vi "Append Page number HF.vi"(0 "PDF Report IN":refnum<class "PDF Report Class.lvclass">, 2 "Header or footer":T1={"Start at page"=1, "Start with #"=1, "Cell Alignment"=1, "Page #"={"Text 1"="", "Text 2"="", "Text 3"=""}, "Font"={"Name"="", "Size"=-1.0, "Color"=0, "Style"={"Bold"=FALSE, "Italic"=FALSE, "Underline"=FALSE, "Strikeout"=FALSE}, "Type"={"Type&direction"=enum."Select", "Embedded"=FALSE, "Encoding"=""}}}, 11 "error in (no error)":errorcluster, 13 "Position":T9) -> (4 "PDF Report OUT":refnum<class "PDF Report Class.lvclass">, 15 "error out":errorcluster)   [LabVIEW 2019, in "Exaprom PDF.lvlib"]
doc: "Appends a <B>page number</B> in a column header (or footer). You can use this polymorphic VI to append a colomn to a header (or footer). The data type you wire to the <B>Header or footer</B> input determines the polymorphic instance to use.\n\nThe header (or footer) can be divided up into three columns. Each column has the same width. The number of header (or footer) that you add determines the number of columns.\n\n<B>FRANÇAIS</B>\nAjoute un <B>numéro de page</B> dans une colonne d'un en-tête (ou d'un pied de page). Vous pouvez utiliser ce VI polymorphique pour ajouter une colonne à un en-tête (ou un pied de page). Le type de variable que vous reliez au terminal <B>Header or footer</B> détermine l'instance polymorphique à utiliser.\n\nL'en-tête (ou le pied de page) peut être divisé en un maximum de trois colonnes. Chaque colonne a la même largeur. Le nombre d'en-têtes (ou de pieds de page) que vous ajoutez détermine le nombre de colonnes.\n\n\n\nVersion 1.1\nDeveloped by Jean-Marc Simard\nCopyright © 2012, Exaprom Inc.\nAll rights reserved.\nLicense: BSD\n\nWith iTextSharp 4.1.6 (http://itextsharp.sourceforge.net)\nunder Mozilla Public License Version 1.1\n(http://www.mozilla.org/MPL/MPL-1.1.html)"
uses:
  Exaprom PDF.lvlib
  LV Class/PDF Report Class/PDF Report Class.lvclass
  Controls/Header, Footer and Watermark Controls/Header or Footer.ctl
  Controls/Header, Footer and Watermark Controls/Header or Footer  Page # cluster.ctl
  Controls/Table Controls/Cell Alignment 20px.ctl
  Controls/Header, Footer and Watermark Controls/Page number.ctl
  Controls/Font Controls/Font complete cluster horizontal.ctl
  Controls/Font Controls/Font size.ctl
  Controls/Font Controls/Font color.ctl
  Controls/Font Controls/Type and encoding.ctl
  Controls/Text Controls/Unicode/Type and run direction.ctl
  LV Class/Header and Footer Class/VIs/Controls/Header Footer cluster V2.ctl
  Controls/Header, Footer and Watermark Controls/Header Footer Type.ctl
  Controls/Header, Footer and Watermark Controls/Header footer horiz alignment.ctl
  Controls/Table Controls/Cell Vertical alignment.ctl
  Controls/Text Controls/Line spacing.ctl
  Controls/Header, Footer and Watermark Controls/Header Footer Line.ctl
  C:/work/niobrara_lv/labview pdf writer fixing/DLL/itextsharp.dll
  DLL/itextsharp.dll
  LV Class/Fonts Class/Font Class.lvclass
  LV Class/Header and Footer Class/Header and Footer Class.lvclass
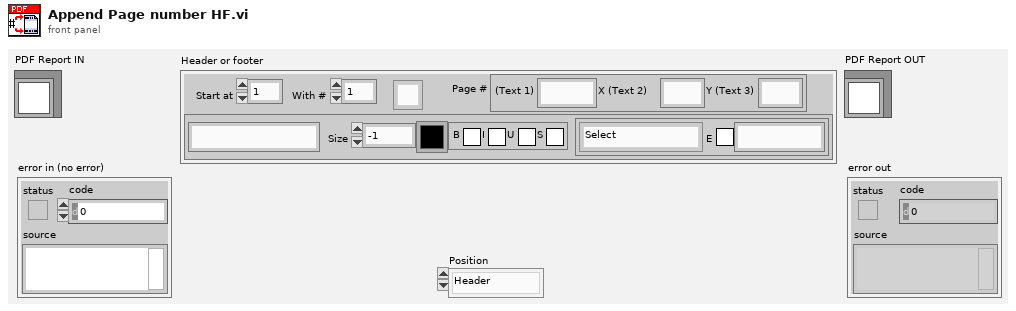
[diagram p1: front panel]
types:
  T1 = typedef "Exaprom PDF.lvlib/Header or Footer  Page # cluster.ctl" = cluster{"Start at page":i32, "Start with #":i32, "Cell Alignment":T2, "Page #":T3, "Font":T4}
  T2 = typedef "Exaprom PDF.lvlib/Cell Alignment 20px.ctl" = u16
  T3 = typedef "Exaprom PDF.lvlib/Page number.ctl" = cluster{"Text 1":string, "Text 2":string, "Text 3":string}
  T4 = typedef "Exaprom PDF.lvlib/Font complete cluster horizontal.ctl" = cluster{"Name":string, "Size":T5, "Color":T6, "Style":cluster{"Bold":bool, "Italic":bool, "Underline":bool, "Strikeout":bool}, "Type":T7}
  T5 = typedef "Exaprom PDF.lvlib/Font size.ctl" = sgl
  T6 = typedef "Exaprom PDF.lvlib/Font color.ctl" = u32
  T7 = typedef "Exaprom PDF.lvlib/Type and encoding.ctl" = cluster{"Type&direction":T8, "Embedded":bool, "Encoding":string}
  T8 = typedef "Exaprom PDF.lvlib/Type and run direction.ctl" = enum16{"Select", "ASCII", "UTF-16", "UTF-16 (default)", "UTF-16 (LTR)", "UTF-16 (RTL)"}
  T9 = typedef "Exaprom PDF.lvlib/Header or Footer.ctl" = enum16{"Header", "Footer"}
  T10 = typedef "Exaprom PDF.lvlib/Header and Footer Class.lvclass/Header Footer cluster V2.ctl" = cluster{"Header or Footer":T9, "Start page":i32, "Start with #":i32, "Type":T11, "Alignment":T12, "Vertical Alignement":T13, "Line spacing":T14, "Image (%)":sgl, "Page #":T3, "Text":string, "Path":string, "Font":T4, "Font refnum":refnum<k24>, "Line":cluster{"Line":T15, "Thickness (points)":sgl, "Colour":T6}, "Vert margin":dbl, "Hyperlink":string}
  T11 = typedef "Exaprom PDF.lvlib/Header Footer Type.ctl" = enum16{"Select", "Text", "Text + hyperlink", "Page number", "Image", "Image + hyperlink"}
  T12 = typedef "Exaprom PDF.lvlib/Header footer horiz alignment.ctl" = enum16{"Left", "Center", "Right"}
  T13 = typedef "Exaprom PDF.lvlib/Cell Vertical alignment.ctl" = enum16{"TOP", "MIDDLE", "BOTTOM"}
  T14 = typedef "Exaprom PDF.lvlib/Line spacing.ctl" = enum16{"Select", "1.0", "1.5", "2.0"}
  T15 = typedef "Exaprom PDF.lvlib/Header Footer Line.ctl" = enum16{"No line", "Horizontal line"}
  T16 = typedef "Exaprom PDF.lvlib/Font complete cluster.ctl" = cluster{"Name":string, "Size":T5, "Color":T6, "Style":cluster{"Bold":bool, "Italic":bool, "Underline":bool, "Strikeout":bool}, "Type":T7}
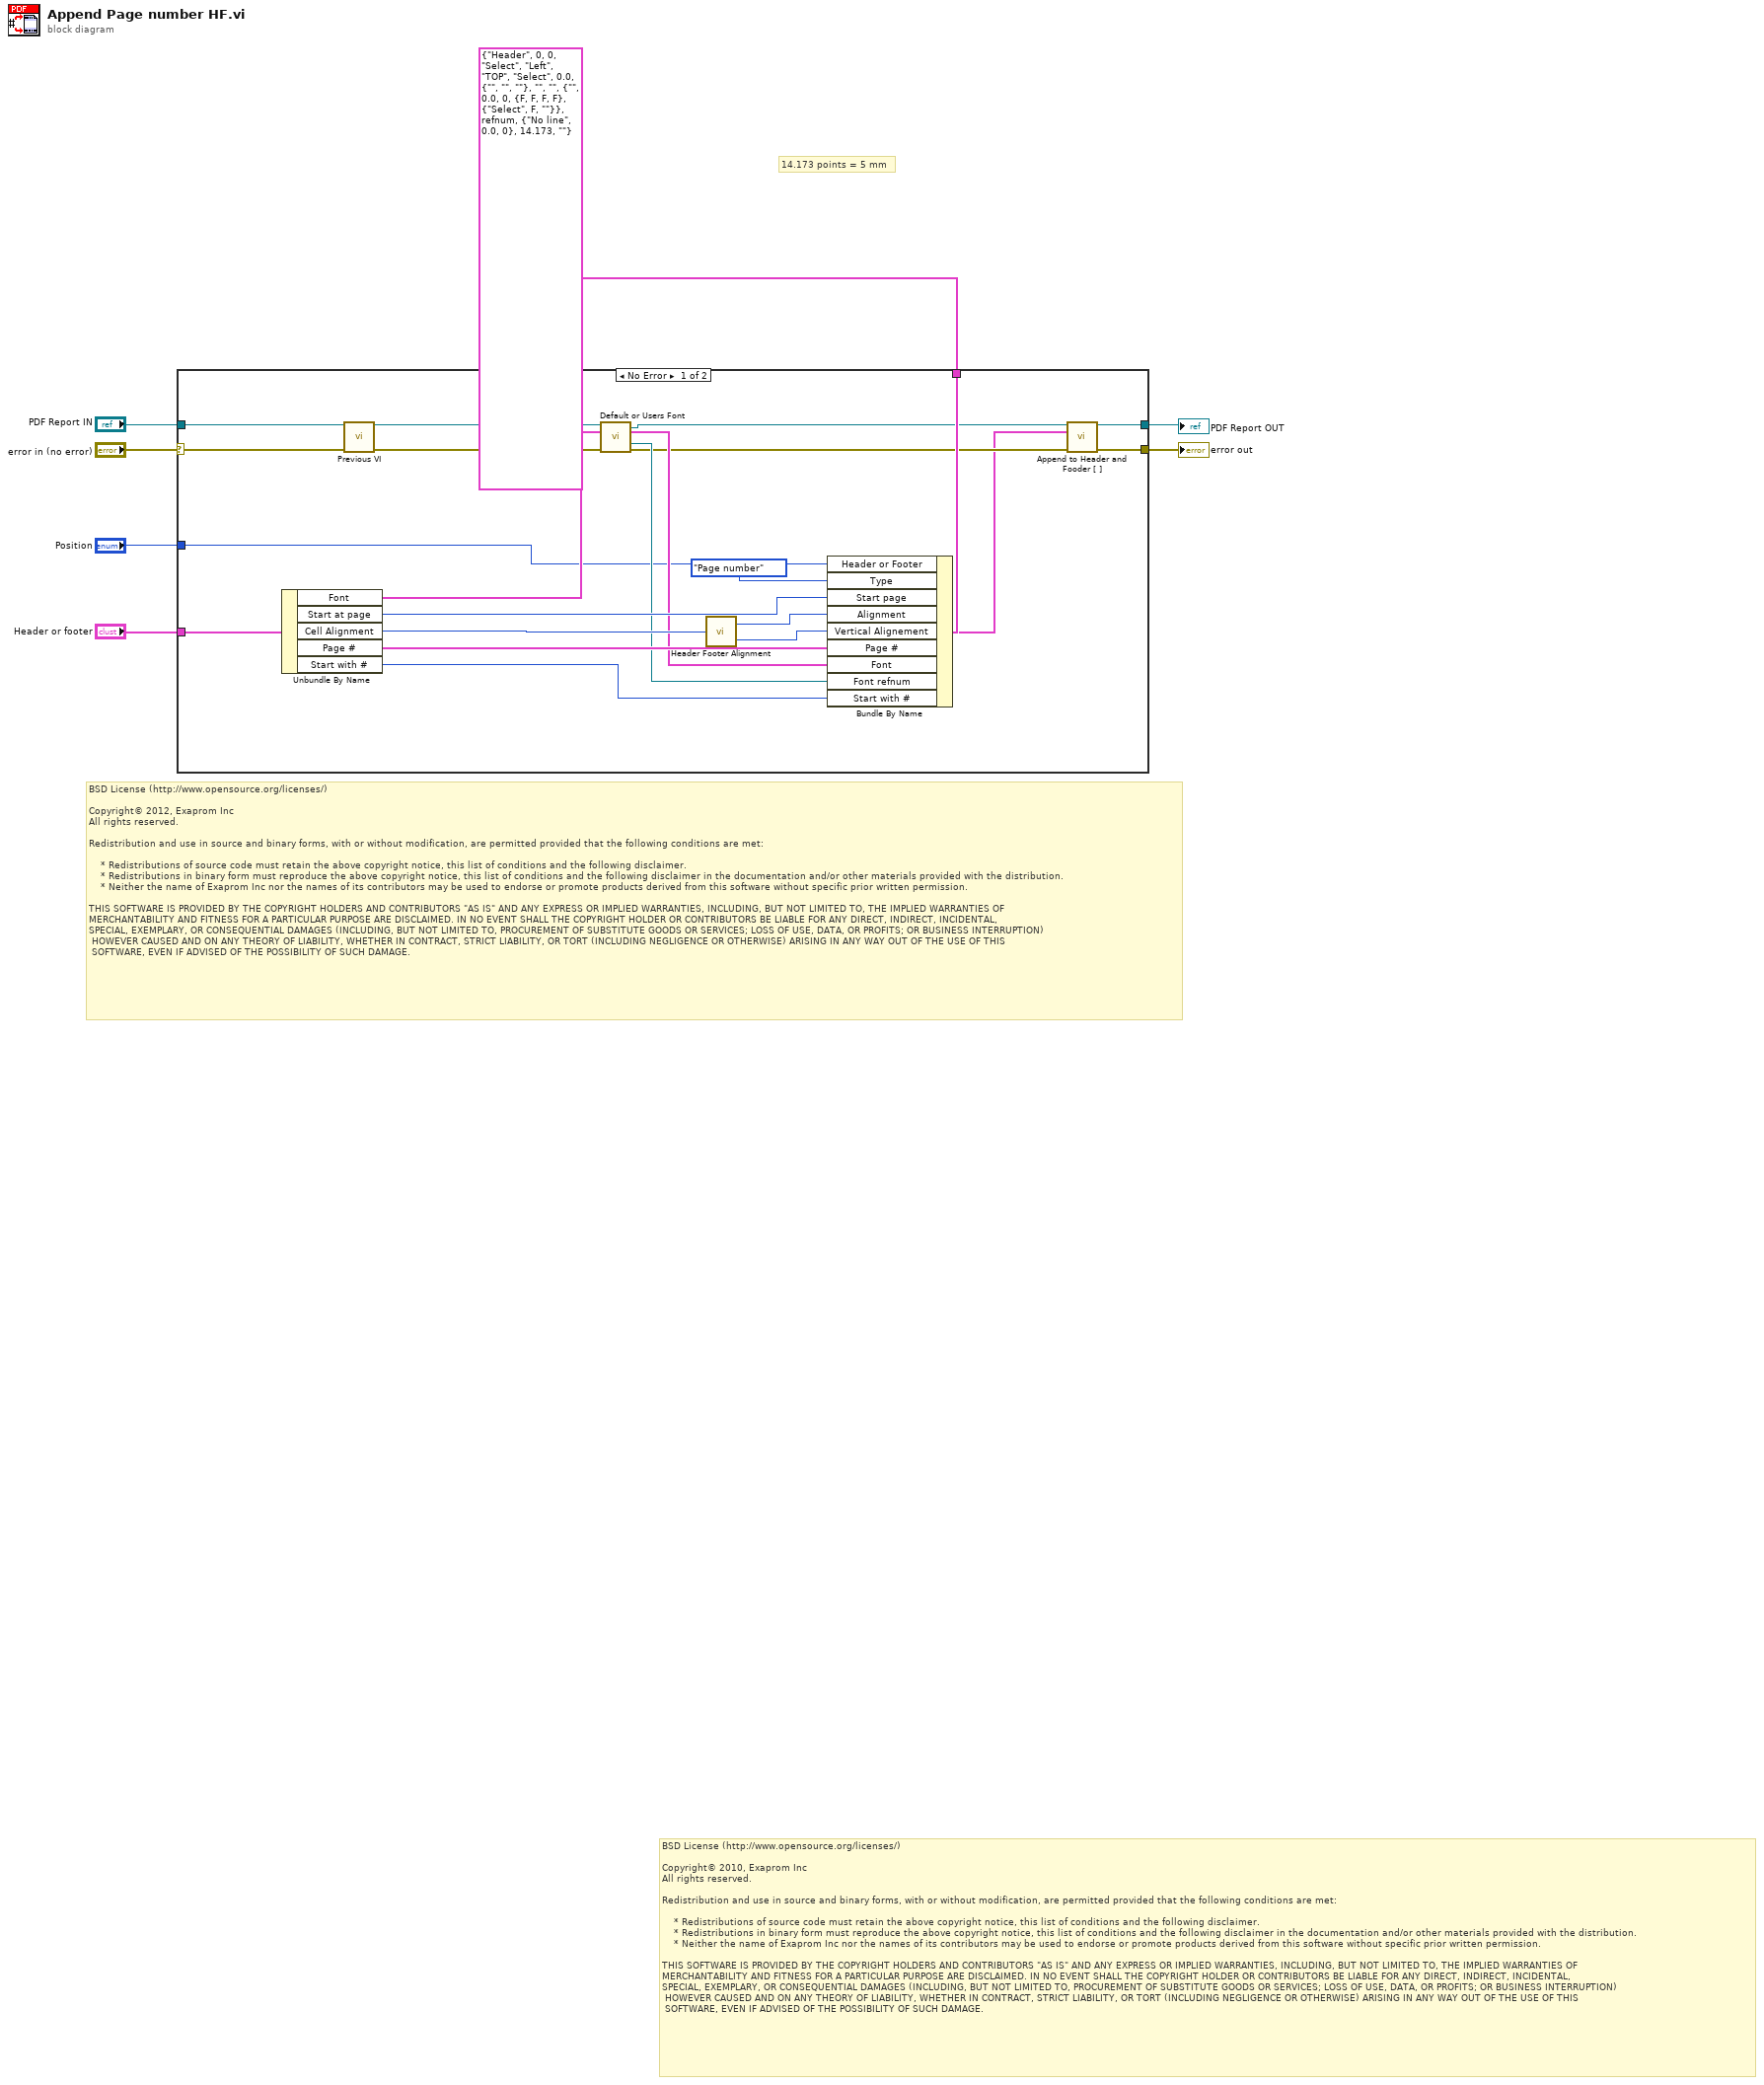
[diagram p0: block diagram]
diagram:
  # "14.173 points = 5 mm"
  # "BSD License (http://www.opensource.org/licenses/)\n\nCopyright© 2012, Exaprom Inc\nAll rights reserved.\n\nRedistribution and use in source and binary forms, with or without modification, are permitted provided that the following conditions are met:\n\n    * Redistributions of source code must retain the above copyright notice, this list of conditions and the following disclaimer.\n    * Redistributions in binary form must reproduce the above copyright notice, this list of conditions and the following disclaimer in the documentation and/or other materials provided with the distribution.\n    * Neither the name of Exaprom Inc nor the names of its contributors may be used to endorse or promote products derived from this software without specific prior written permission.\n\nTHIS SOFTWARE IS PROVIDED BY THE COPYRIGHT HOLDERS AND CONTRIBUTORS \"AS IS\" AND ANY EXPRESS OR IMPLIED WARRANTIES, INCLUDING, BUT NOT LIMITED TO, THE IMPLIED WARRANTIES OF \nMERCHANTABILITY AND FITNESS FOR A PARTICULAR PURPOSE ARE DISCLAIMED. IN NO EVENT SHALL THE COPYRIGHT HOLDER OR CONTRIBUTORS BE LIABLE FOR ANY DIRECT, INDIRECT, INCIDENTAL,\nSPECIAL, EXEMPLARY, OR CONSEQUENTIAL DAMAGES (INCLUDING, BUT NOT LIMITED TO, PROCUREMENT OF SUBSTITUTE GOODS OR SERVICES; LOSS OF USE, DATA, OR PROFITS; OR BUSINESS INTERRUPTION)\n HOWEVER CAUSED AND ON ANY THEORY OF LIABILITY, WHETHER IN CONTRACT, STRICT LIABILITY, OR TORT (INCLUDING NEGLIGENCE OR OTHERWISE) ARISING IN ANY WAY OUT OF THE USE OF THIS\n SOFTWARE, EVEN IF ADVISED OF THE POSSIBILITY OF SUCH DAMAGE."
  # "BSD License (http://www.opensource.org/licenses/)\n\nCopyright© 2010, Exaprom Inc\nAll rights reserved.\n\nRedistribution and use in source and binary forms, with or without modification, are permitted provided that the following conditions are met:\n\n    * Redistributions of source code must retain the above copyright notice, this list of conditions and the following disclaimer.\n    * Redistributions in binary form must reproduce the above copyright notice, this list of conditions and the following disclaimer in the documentation and/or other materials provided with the distribution.\n    * Neither the name of Exaprom Inc nor the names of its contributors may be used to endorse or promote products derived from this software without specific prior written permission.\n\nTHIS SOFTWARE IS PROVIDED BY THE COPYRIGHT HOLDERS AND CONTRIBUTORS \"AS IS\" AND ANY EXPRESS OR IMPLIED WARRANTIES, INCLUDING, BUT NOT LIMITED TO, THE IMPLIED WARRANTIES OF \nMERCHANTABILITY AND FITNESS FOR A PARTICULAR PURPOSE ARE DISCLAIMED. IN NO EVENT SHALL THE COPYRIGHT HOLDER OR CONTRIBUTORS BE LIABLE FOR ANY DIRECT, INDIRECT, INCIDENTAL,\nSPECIAL, EXEMPLARY, OR CONSEQUENTIAL DAMAGES (INCLUDING, BUT NOT LIMITED TO, PROCUREMENT OF SUBSTITUTE GOODS OR SERVICES; LOSS OF USE, DATA, OR PROFITS; OR BUSINESS INTERRUPTION)\n HOWEVER CAUSED AND ON ANY THEORY OF LIABILITY, WHETHER IN CONTRACT, STRICT LIABILITY, OR TORT (INCLUDING NEGLIGENCE OR OTHERWISE) ARISING IN ANY WAY OUT OF THE USE OF THIS\n SOFTWARE, EVEN IF ADVISED OF THE POSSIBILITY OF SUCH DAMAGE."
  n1 = case shown="No Error" "error in (no error)" {
    selector: "error in (no error)" -> [w22 w31]
    tunnel: "PDF Report IN" -> [w23 w30]
    tunnel: "Position" -> [w16 _]
    tunnel: [w15 w30] -> w2
    tunnel: [w14 w31] -> w3
    tunnel: "Header or footer" -> [w21 _]
    tunnel: T10 {"Header or Footer"=enum."Header", "Start page"=0, "Start with #"=0, "Type"=enum."Select", "Alignment"=enum."Left", "Vertical Alignement"=enum."TOP", "Line spacing"=enum."Select", "Image (%)"=0.0, "Page #"={"Text 1"="", "Text 2"="", "Text 3"=""}, "Text"="", "Path"="", "Font"={"Name"="", "Size"=0.0, "Color"=0, "Style"={"Bold"=FALSE, "Italic"=FALSE, "Underline"=FALSE, "Strikeout"=FALSE}, "Type"={"Type&direction"=enum."Select", "Embedded"=FALSE, "Encoding"=""}}, "Font refnum"=refnum, "Line"={"Line"=enum."No line", "Thickness (points)"=0.0, "Colour"=0}, "Vert margin"=14.173, "Hyperlink"=""} ("Cluster") -> [w17 _]
    frame No Error {
      n2 = Unbundle By Name(w21) -> ("Font"=w20:T4, "Start at page"=w29:i32, "Cell Alignment"=w28:T2, "Page #"=w25:T3, "Start with #"=w10:i32)
      n3 = call "Previous VI.vi"("PDF Report IN"=w23, "error in (no error)"=w22) -> ("PDF Report OUT"=w8:refnum<class "PDF Report Class.lvclass">, "error out"=w9:errorcluster)  [unwired: 12 out]
      n4 = call "Default or Users Font.vi"("PDF Report"=w8, "Font"=w20, "error in (no error)"=w9) -> ("PDF Report duplicate"=w12:refnum<class "PDF Report Class.lvclass">, "Font OUT"=w19:T16, "Font Ref"=w18:refnum<k24>, "error out"=w13:errorcluster)  [unwired: 7 in, 2 out]
      n5 = call "Header Footer Alignment.vi"("Cell Alignment"=w28) -> ("Vertical Alignement"=w26:T13, "Horizontal Alignment"=w27:T12)  [unwired: 2 out]
      n6 = Bundle By Name(cluster=w17, "Header or Footer"=w16, "Type"=Header_Footer_Type."Page number", "Start page"=w29, "Alignment"=w27, "Vertical Alignement"=w26, "Page #"=w25, "Font"=w19, "Font refnum"=w18, "Start with #"=w10) -> (w11:T10)
      n7 = call "Append to Header and Fooder [ ].vi"("PDF Report IN"=w12, "Header and Footer"=w11, "error in (no error)"=w13) -> ("PDF Report OUT"=w15:refnum<class "PDF Report Class.lvclass">, "error out"=w14:errorcluster)  [unwired: 11 in]
    }
    frame Error {
    }
  }
  "PDF Report OUT" <- w2
  "error out" <- w3
